vi "Target.vi"() -> ()   [LabVIEW 2025]
uses:
  <vilib>/Platform/TimedLoop/XDataNode/timing_clust.ctl
  <vilib>/Platform/TimedLoop/XDataNode/nitl_modes.ctl
  <vilib>/Platform/TimedLoop/XDataNode/wakeup.ctl
  <vilib>/eio/utilities/niEioResolveVilibRelativePath.vi
  <vilib>/rvi/interface/RandomDataEmulation/niFpgaRandomDataHandleErrors.vi
  <vilib>/rvi/Emulation/niFpgaSctlEmulationGetInTimedLoop.vi
  <vilib>/rvi/Emulation/niFpgaEmulationReportErrorSimple.vi
  <vilib>/rvi/Emulation/niFpgaGetClockAttributes.vi
  <vilib>/rvi/Emulation/niFpgaCriticalErrorInLSC.vi
  <vilib>/rvi/interface/RandomDataEmulation/nirviRandomDataMultiElementFPGAFIFO.vi
  <instcachedir>/0/nirviRandomDataMultiElementFPGAFIFO_BE2FF10D3D6E420AB0291A02835C249E.lvgen/nirviRandomDataMultiElementFPGAFIFO_BE2FF10D3D6E420AB0291A02835C249E_001.vi
  <vilib>/rvi/linearAlgebra/MatrixMultiply/simVIs/SubVI/nifxpla_MatrixMultiply_SimMatrixSizes.vi
  <vilib>/rvi/linearAlgebra/MatrixMultiply/simVIs/SubVI/nifxpla_MatrixMultiply_Sim4WireAdapterVector.vi
  <vilib>/rvi/linearAlgebra/MatrixMultiply/simVIs/SubVI/nifxpla_MatrixMultiply_SimFrameHandShake.vi
  <vilib>/rvi/linearAlgebra/MatrixMultiply/simVIs/SubVI/nifxpla_MatrixMultiply_SimEndlessCounter.vi
  <vilib>/rvi/linearAlgebra/MatrixMultiply/simVIs/SubVI/nifxpla_MatrixMultiply_SimVectorDataBuffer.vi
  <vilib>/rvi/ClientSDK/Core/DevComputerLib/Private/Multiply(dfxp64).vi
  <vilib>/rvi/ClientSDK/Core/DevComputerLib/Private/Dfxp128ToDfxp256.vi
  <vilib>/rvi/ClientSDK/Core/DevComputerLib/Private/Add(dfxp256).vi
  <vilib>/rvi/ClientSDK/Core/DevComputerLib/Private/Subtract(dfxp256).vi
  <vilib>/rvi/ClientSDK/Core/DevComputerLib/Private/ToDfxp64(dfxp256).vi
  <vilib>/rvi/DataTransferAndStorage/Container/XNode/niFpgaContainer.xnode
  <vilib>/rvi/interface/RandomDataEmulation/nirviRandomDataFpgaReadWriteTemplate.vi
  <vilib>/platform/TimedLoop/XDataNode/XDataNode.xnode
  <vilib>/rvi/interface/RandomDataEmulation/nirviRandomDataFpgaMultiElementTemplate.vi
  <vilib>/rvi/linearAlgebra/MatrixMultiply/XNode/nifxpla_MatrixMultiply.xnode
  <vilib>/rvi/linearAlgebra/MatrixMultiply/simVIs/nifxpla_MatrixMultiply_SimTemplateEinEout.vi
  <vilib>/rvi/linearAlgebra/MatrixMultiply/simVIs/nifxpla_MatrixMultiply_SimTemplateEinVout.vi
  <vilib>/rvi/linearAlgebra/MatrixMultiply/simVIs/nifxpla_MatrixMultiply_SimTemplateVinEout.vi
  <vilib>/rvi/linearAlgebra/MatrixMultiply/simVIs/nifxpla_MatrixMultiply_SimTemplateVinVout.vi
  <vilib>/Platform/TimedLoop/XDataNode/XDNodeRunTimeDep.lvlib
panel:
  out "Array 2.1":fxp<+/-,32,16>[](array[numeric])
  out "Array 1.2":fxp<+/-,32,16>[](array[numeric])
  out "Array 2":fxp<+/-,32,16>[](array[numeric])
  out "Array 1":fxp<+/-,32,16>[](array[numeric])
  out "element 4":fxp<+/-,32,16>
  out "element 3":fxp<+/-,32,16>
  out "element 2":fxp<+/-,32,16>
  out "element":fxp<+/-,32,16>
  out "interleaved array 2":fxp<+/-,32,16>[](array[numeric])
  out "interleaved array":fxp<+/-,32,16>[](array[numeric])
  out "Case Number":i16
  out "Numeric":i32
  out "appended array 2":fxp<+/-,32,16>[](array[numeric])
  out "appended array":fxp<+/-,32,16>[](array[numeric])
  out "cr":fxp<+/-,32,16>[](array[numeric])
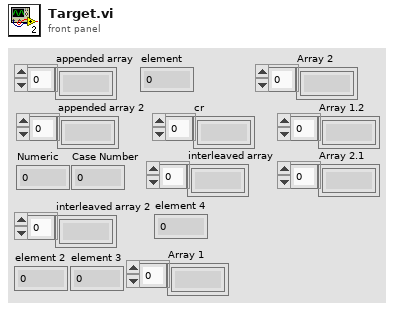
[diagram p1: front panel]
types:
  T1 = typedef "XDNodeRunTimeDep.lvlib/timing_clust.ctl" = cluster{"Expected End [f-1]":u64, "Actual End [f-1]":u64, "Finished Late? [f-1]":bool, "Expected End [i-1]":u64, "Actual End [i-1]":u64, "Finished Late? [i-1]":bool, "Expected Start [i]":u64, "Actual Start [i]":u64, "Expected Start [f]":u64, "Actual Start [f]":u64, "Source Name":string, "Structure Name":string, "Period":i64, "Deadline":i64, "Offset":i64, "Start":i64, "Priority":i32, "Timeout":i32, "Mode":T2, "Wakeup Reason":T3, "Error":errorcluster, "Source Type":string, "Secondary Source Type":string, "Global End Time":u64, "Global Start Time":u64, "Frame Duration":u64, "Iteration Duration":u64, "Assigned CPU":i32, "I/O Scan Engine Mode":u32}
  T2 = typedef "XDNodeRunTimeDep.lvlib/nitl_modes.ctl" = enum32{"No Change", "Process missed periods, maintain original phase", "Discard missed periods, maintain original phase", "Process missed periods, ignore original phase", "Discard missed periods, ignore original phase"}
  T3 = typedef "XDNodeRunTimeDep.lvlib/wakeup.ctl" = enum32{"Normal", "Aborted", "Asynchronous wakeup", "Timing source error", "Timed loop error", "Timeout"}
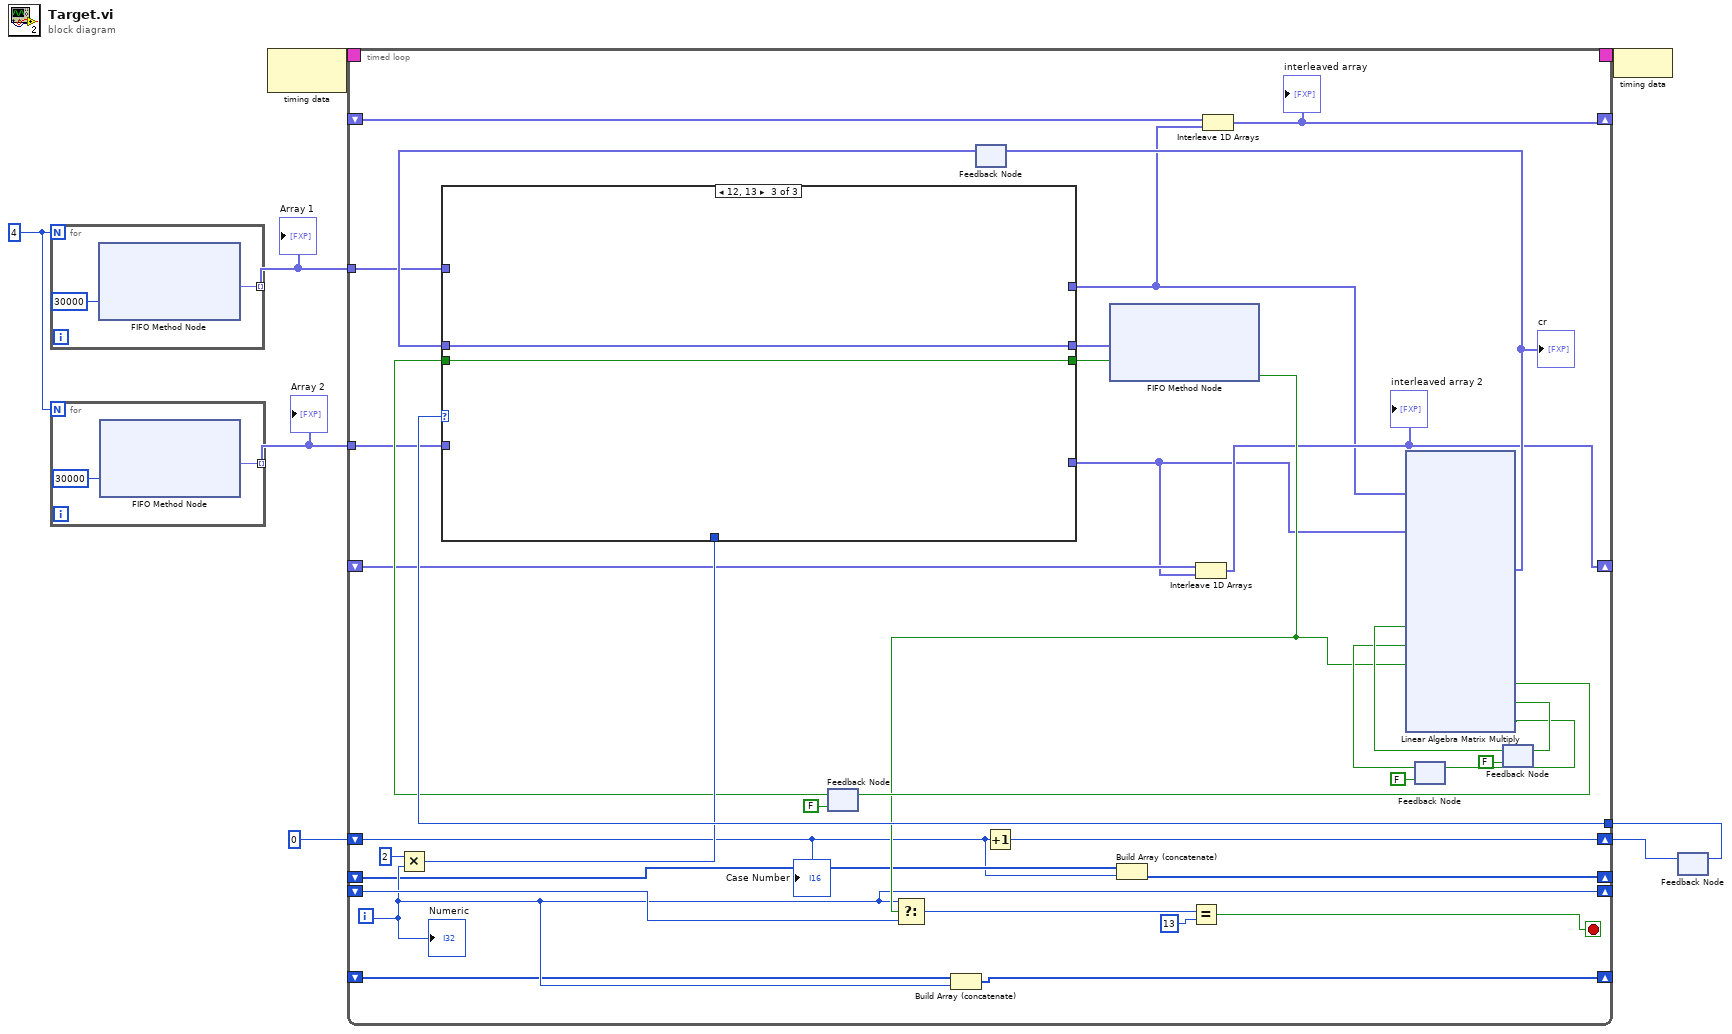
[diagram p0: block diagram]
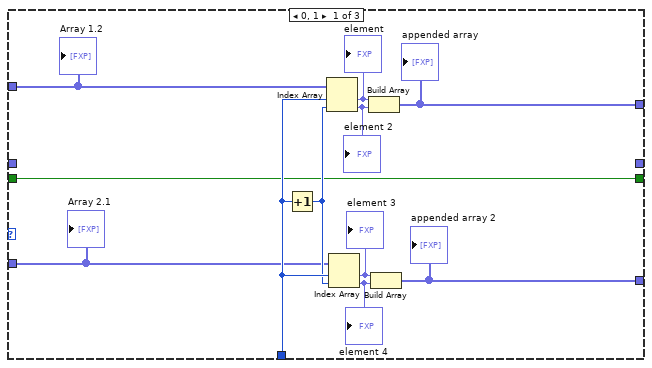
[diagram p2: hidden frame]
diagram:
  w3 = 4
  n1 = for {
    N: w3 -> [_]
    tunnel: [w10] -> w2 mode=indexing
    n2 = xnode ("FIFO Method Node")("Timeout"=30000) -> ("Element"=w10:fxp<+/-,32,16>)  [unwired: 1 in, 2 out]
  }
  "Array 1" <- w2
  n3 = for {
    N: w3 -> [_]
    tunnel: [w12] -> w1 mode=indexing
    n4 = xnode ("FIFO Method Node")("Timeout"=30000) -> ("Element"=w12:fxp<+/-,32,16>)  [unwired: 1 in, 2 out]
  }
  "Array 2" <- w1
  n5 = node-c288() -> (w8:T1)  [unwired: 1 in]
  n6 = feedback #1() -> (w4:i16)  [unwired: 1 in]
  n7 = timed-loop {
    timing: w8 -> [_]
    timing-out: [_] -> w7
    shift-right: [w48] -> w5
    shift-left: i16 0 -> [w13]
    tunnel: w4 -> [w47]
    shift-right: [w18] -> _
    shift-left: _ -> [w36]
    tunnel: w2 -> [w29]
    tunnel: w1 -> [w28]
    shift-right: [w22] -> _
    shift-left: _ -> [w23]
    shift-right: [w21] -> _
    shift-left: _ -> [w24]
    shift-right: [w16] -> _
    shift-left: _ -> [w17]
    shift-right: [w14] -> _
    shift-left: _ -> [w15]
    i -> [w18]
    stop <- w33 stop-if-true
    n8 = Multiply(x=2, y=w18) -> (x*y=w45:i32)
    n9 = feedback #2(FALSE ("output valid")) -> (w31:bool)
    n10 = Build Array (concatenate)(w17, w18) -> (w16:i32[])
    n11 = feedback #3() -> (w43:fxp<+/-,32,16>[])  [unwired: 1 in]
    n12 = case shown="12, 13" w47 {
      tunnel: [w55 _ _] -> w20
      tunnel: [w54 _ _] -> w19
      tunnel: w45 -> [w53 _ _]
      tunnel: w43 -> [_ _ w62]
      tunnel: w31 -> [w49 w60 w61]
      tunnel: w29 -> [w51 _ _]
      tunnel: w28 -> [w50 _ _]
      tunnel: [_ _ w62] -> w26
      tunnel: [w49 w60 w61] -> w25
      frame 0, 1 {
        n13 = Increment(x=w53) -> (x+1=w52:i32)
        n14 = Index Array(array=w51, index #1=w53, index #2=w52) -> (element #1=w57:fxp<+/-,32,16>, element #2=w56:fxp<+/-,32,16>)
        "element" <- w57
        "element 2" <- w56
        n15 = Index Array(array=w50, index #1=w53, index #2=w52) -> (element #1=w59:fxp<+/-,32,16>, element #2=w58:fxp<+/-,32,16>)
        "element 3" <- w59
        "element 4" <- w58
        n16 = Build Array(w57, w56) -> (w55:fxp<+/-,32,16>[])
        "appended array" <- w55
        n17 = Build Array(w59, w58) -> (w54:fxp<+/-,32,16>[])
        "appended array 2" <- w54
        "Array 1.2" <- w51
        "Array 2.1" <- w50
      }
      frame 2, Default {
      }
      frame 12, 13 {
      }
    }
    n18 = Increment(x=w13) -> (x+1=w48:i16)
    n19 = xnode ("FIFO Method Node")("Element"=w26, "Input Valid"=w25) -> ("Ready for Input"=w27:bool)  [unwired: 1 in, 1 out]
    n20 = Select(t=w18, s=w27, f=w36) -> (s? t:f=w35:i32)
    n21 = Build Array (concatenate)(w15, w13) -> (w14:i16[])
    n22 = Equal?(x=w35, y=13) -> (x = y?=w33:bool)
    n23 = Interleave 1D Arrays(w24, w19) -> (w21:fxp<+/-,32,16>[])
    "interleaved array 2" <- w21
    n24 = Interleave 1D Arrays(w23, w20) -> (w22:fxp<+/-,32,16>[])
    "interleaved array" <- w22
    n25 = feedback #4(FALSE ("ready for b")) -> (w39:bool)
    n26 = feedback #5(FALSE ("ready for a")) -> (w41:bool)
    n27 = xnode ("Linear Algebra Matrix Multiply")("ar"=w20, "br"=w19, "a valid"=w41, "b valid"=w39, "ready for output (T)"=w27) -> ("cr"=w44:fxp<+/-,32,16>[], "output valid"=w32:bool, "ready for a"=w42:bool, "ready for b"=w40:bool)  [unwired: 2 in, 2 out]
    "cr" <- w44
    n28 = feedback-in #2(w32) -> ()
    n29 = feedback-in #3(w44) -> ()
    n30 = feedback-in #4(w40) -> ()
    n31 = feedback-in #5(w42) -> ()
    "Numeric" <- w18
    "Case Number" <- w13
  }
  n32 = node-c288(w7) -> ()
  n33 = feedback-in #1(w5) -> ()
